vi "Camera xyhl 2P.vi"(10 "tableau":u8[](array[numeric])) -> (2 "Indications pokaenmon":T1)   [LabVIEW 2013]
panel:
  out "sign":string
  out "h":string
  out "L":string
  out "y":string
  out "x":string
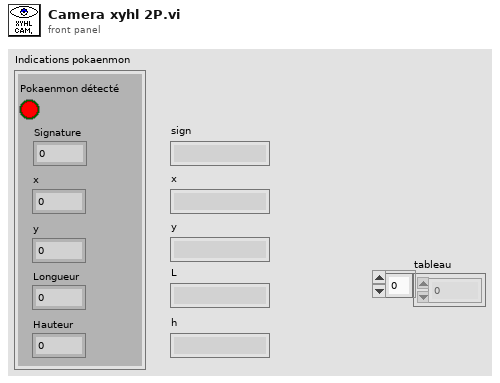
[diagram p1: front panel]
types:
  T1 = cluster{"Pokaenmon détecté":bool, "Signature":u32, "x":dbl, "y ":dbl, "Longueur":dbl, "Hauteur":dbl}
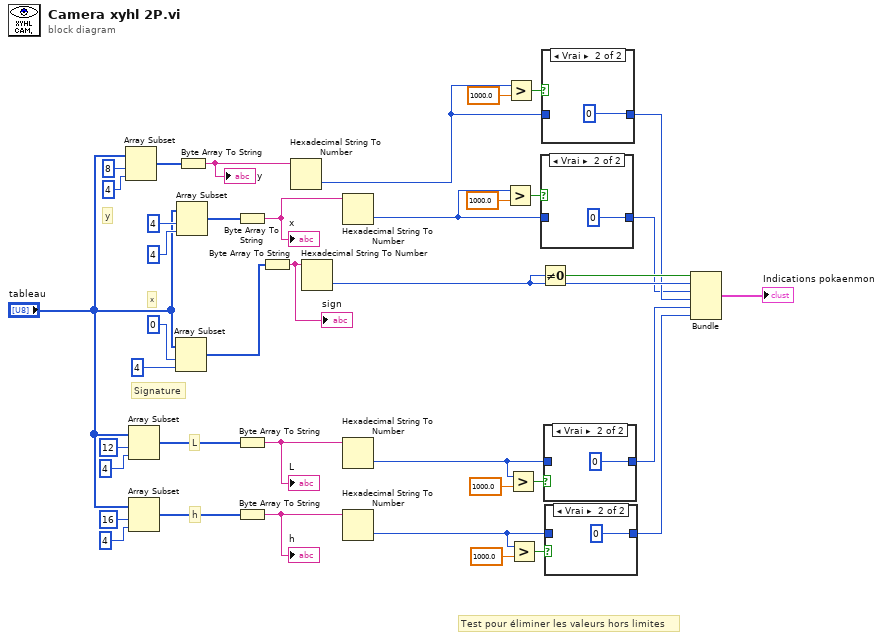
[diagram p0: block diagram]
diagram:
  # "Test pour éliminer les valeurs hors limites"
  # "h"
  # "L"
  # "y"
  # "x"
  # "Signature"
  n1 = Array Subset(array="tableau", index=8 ("offset (0)"), length=4 ("longueur (reste)")) -> (w31:u8[])
  n2 = Array Subset(array="tableau", index=12 ("offset (0)"), length=4 ("longueur (reste)")) -> (w32:u8[])
  n3 = Array Subset(array="tableau", index=16 ("offset (0)"), length=4 ("longueur (reste)")) -> (w33:u8[])
  n4 = Array Subset(array="tableau", index=0 ("offset (0)"), length=4 ("longueur (reste)")) -> (w17:u8[])
  n5 = Array Subset(array="tableau", index=4 ("offset (0)"), length=4 ("longueur (reste)")) -> (w30:u8[])
  n6 = Byte Array To String(unsigned byte array=w31) -> (string=w35:string)
  "y" <- w35
  n7 = Byte Array To String(unsigned byte array=w30) -> (string=w36:string)
  "x" <- w36
  n8 = Byte Array To String(unsigned byte array=w32) -> (string=w34:string)
  "L" <- w34
  n9 = Byte Array To String(unsigned byte array=w33) -> (string=w37:string)
  "h" <- w37
  n10 = Byte Array To String(unsigned byte array=w17) -> (string=w40:string)
  "sign" <- w40
  n11 = Hexadecimal String To Number(string=w35) -> (number=w3:u32)  [unwired: 2 in, 1 out]
  n12 = Hexadecimal String To Number(string=w40) -> (number=w39:u32)  [unwired: 2 in, 1 out]
  n13 = Hexadecimal String To Number(string=w36) -> (number=w1:u32)  [unwired: 2 in, 1 out]
  n14 = Hexadecimal String To Number(string=w34) -> (number=w5:u32)  [unwired: 2 in, 1 out]
  n15 = Hexadecimal String To Number(string=w37) -> (number=w7:u32)  [unwired: 2 in, 1 out]
  n16 = Greater?(x=w1, y=1000.0) -> (0:w16:bool)
  n17 = Greater?(x=w3, y=1000.0) -> (0:w14:bool)
  n18 = Greater?(x=w5, y=1000.0) -> (0:w12:bool)
  n19 = Greater?(x=w7, y=1000.0) -> (0:w10:bool)
  n20 = Not Equal To 0?(x=w39) -> (x != 0?=w19:bool)
  n21 = case shown="Vrai" w16 {
    tunnel: [w41 0] -> w2
    tunnel: w1 -> [w41 _]
    frame False {
    }
    frame True {
    }
  }
  n22 = case shown="Vrai" w14 {
    tunnel: [w43 0] -> w4
    tunnel: w3 -> [w43 _]
    frame False {
    }
    frame True {
    }
  }
  n23 = case shown="Vrai" w12 {
    tunnel: [w45 0] -> w6
    tunnel: w5 -> [w45 _]
    frame False {
    }
    frame True {
    }
  }
  n24 = case shown="Vrai" w10 {
    tunnel: [w47 0] -> w8
    tunnel: w7 -> [w47 _]
    frame False {
    }
    frame True {
    }
  }
  n25 = Bundle(w19, w39, w2, w4, w6, w8) -> (→"Indications pokaenmon":cluster{bool, u32, u32, u32, u32, u32})  [unwired: 1 in]
